vi "Test Zj(r,t=const).vi"() -> ()   [LabVIEW 2013, in "Zernike Polynome.lvlib"]
doc: "This VI is used to thest the radial behaviour of Zj(r,theta=const)."
uses:
  Zernike Polynome.lvlib
  <vilib>/Utility/error.llb/DialogType.ctl
panel:
  out "j":i32
  out "Zj(r,t=const)":cluster{i32, dbl, dbl[]}(graph)
  in  "Nof Points":i32
  in  "j (1)":i32=1
  in  "theta":dbl
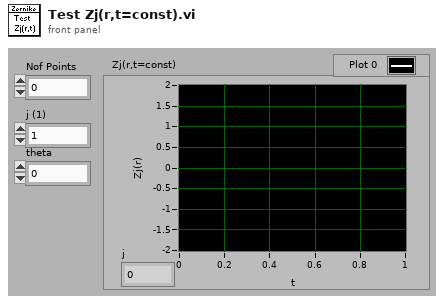
[diagram p1: front panel]
types:
  T1 = typedef "DialogType.ctl" = u16
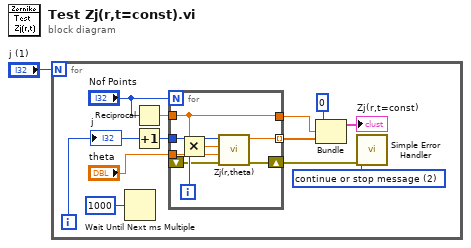
[diagram p0: block diagram]
diagram:
  n1 = for {
    N: "j (1)" -> [_]
    i -> [w9]
    w7 = T1 2 items=["no dialog", "OK message", "continue or stop message", "OK message + warnings", "continue/stop + warnings"] ("type of dialog (OK msg:1)")
    n2 = Wait Until Next ms Multiple(millisecond multiple=u32 1000) -> ()  [unwired: 1 out]
    n3 = Reciprocal(x="Nof Points") -> (1/x=w11:dbl)
    n4 = Increment(x=w9) -> (x+1=w6:i32)
    n5 = for {
      N: "Nof Points" -> [_]
      tunnel: "theta" -> [w20]
      tunnel: w6 -> [w19]
      tunnel: w11 -> [w15]
      shift-right: [w21] -> w10
      shift-left: _ -> [w17]
      tunnel: [w15] -> w4
      tunnel: [w14] -> w5 mode=indexing
      i -> [w18]
      n6 = Multiply(x=w15, y=w18) -> (x*y=w16:dbl)
      n7 = call "Zj(r,theta).vi"("error in (no error)"=w17, "theta"=w20, "r"=w16, "j (1)"=w19) -> ("error out"=w21:errorcluster, "Zj(r,theta)"=w14:dbl)  [unwired: 2 out]
    }
    n8 = Bundle(0, w4, w5) -> (→"Zj(r,t=const)":cluster{i32, dbl, dbl[]})  [unwired: 1 in]
    n9 = call <vilib>:"Simple Error Handler.vi"("type of dialog (OK msg:1)"=w7, "error in (no error)"=w10) -> ()  [unwired: 3 in, 5 out]
    "j" <- w9
  }
